vi "subAcquisition_UpdateZ.vi"(6 "Ref":T1, 7 "z":dbl, 8 "error in":errorcluster, 11 "TiCtrl ref in":refnum<vi>) -> (0 "error out":errorcluster, 3 "TiCtrl ref out":refnum<vi>)   [LabVIEW 2015]
panel:
  # "Move z, and update front panel"
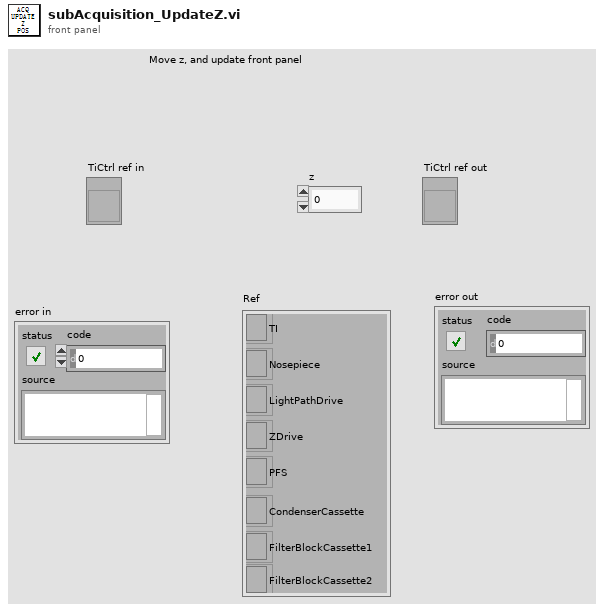
[diagram p1: front panel]
types:
  T1 = cluster{"TI":refnum<k7>, "Nosepiece":refnum<k7>, "LightPathDrive":refnum<k7>, "ZDrive":refnum<k7>, "PFS":refnum<k7>, "CondenserCassette":refnum<k7>, "FilterBlockCassette1":refnum<k7>, "FilterBlockCassette2":refnum<k7>}
  T2 = cluster{"Obj":u16, "Cube Bottom":u16, "Cube Top":u16, "PFS-Ctrl":cluster{"PFS IO":bool, "PSF Err":bool, "PSF Pos":u32}, "Z-Ctrl":cluster{"Z-pos":dbl, "Home":bool, "Sensitivity":u8}, "Condenser":u16, "Lightpath":enum32{"EYE", "L100", "R100", "L80"}}
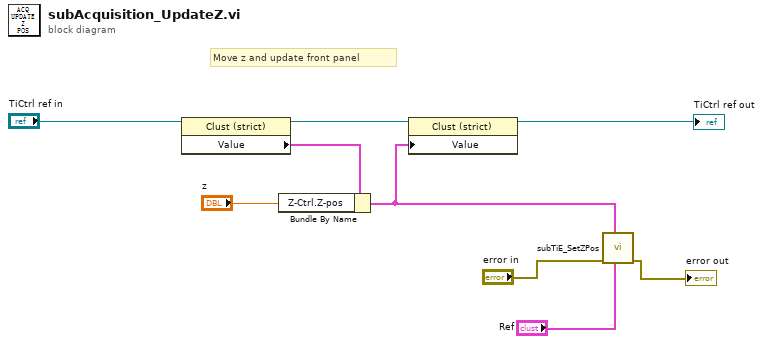
[diagram p0: block diagram]
diagram:
  # "Move z and update front panel"
  n1 = property class="Clust (strict)"(reference="TiCtrl ref in") -> (reference out=w6:refnum<vi>, "Value"=w7:T2)  [unwired: 1 in, 1 out]
  n2 = Bundle By Name(cluster=w7, "Z-Ctrl.Z-pos"="z") -> (w4:T2)
  n3 = property class="Clust (strict)"(reference=w6, "Value"=w4) -> (reference out=→"TiCtrl ref out":refnum<vi>)  [unwired: 1 in, 1 out]
  n4 = call "subTiE_SetZPos.vi"("Ref"="Ref", "TI-Ctrl"=w4, "error in"="error in") -> ("error out"=→"error out":errorcluster)  [unwired: 8 in]
